vi "bytesFind.vi"(9 "find bytes":u8[](array[numeric]), 11 "log":u8[](array[numeric])) -> (0 "parsing error":bool, 1 "deleted portion":u8[](array[numeric]), 3 "rest of the log":u8[](array[numeric]))   [LabVIEW 2023]
panel:
  out "errors":bool[](array[boolean])
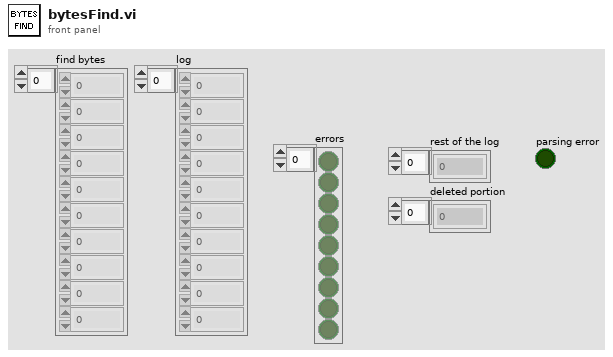
[diagram p1: front panel]
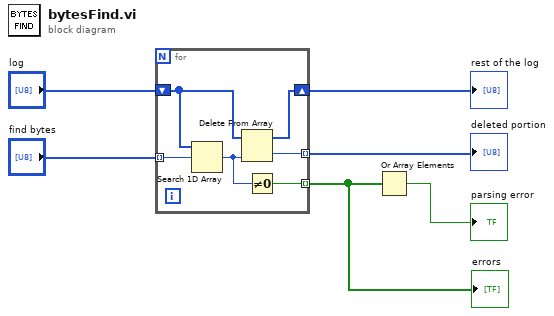
[diagram p0: block diagram]
diagram:
  n1 = for {
    tunnel: "find bytes" -> [w12] mode=indexing
    shift-right: [w10] -> w3
    shift-left: "log" -> [w11]
    tunnel: [w8] -> w6 mode=indexing
    tunnel: [w7] -> w2 mode=indexing
    n2 = Search 1D Array(1D array=w11, element=w12) -> (index of element=w9:i32)  [unwired: 1 in]
    n3 = Delete From Array(array=w11, index=w9) -> (deleted portion=w7:u8, array with subset deleted=w10:u8[])  [unwired: 1 in]
    n4 = Not Equal To 0?(x=w9) -> (x != 0?=w8:bool)
  }
  "rest of the log" <- w3
  "deleted portion" <- w2
  "errors" <- w6
  n5 = Or Array Elements(Boolean array=w6) -> (logical OR=→"parsing error":bool)
